vi "AFM_Driver_Manager.CreateAbort.vi"(8 "error in (no error)":errorcluster, 11 "AFM_Driver_Manager in":refnum<class "AFM_Driver_Manager.lvclass">) -> (0 "error out":errorcluster, 3 "AFM_Driver_Manager out":refnum<class "AFM_Driver_Manager.lvclass">)   [LabVIEW 2019, in "AFM_Driver_Manager.lvclass"]
uses:
  AFM_Driver_Manager.lvclass
  AFM_Driver_Manager.lvclass/AFM_Driver_Manager.ctl
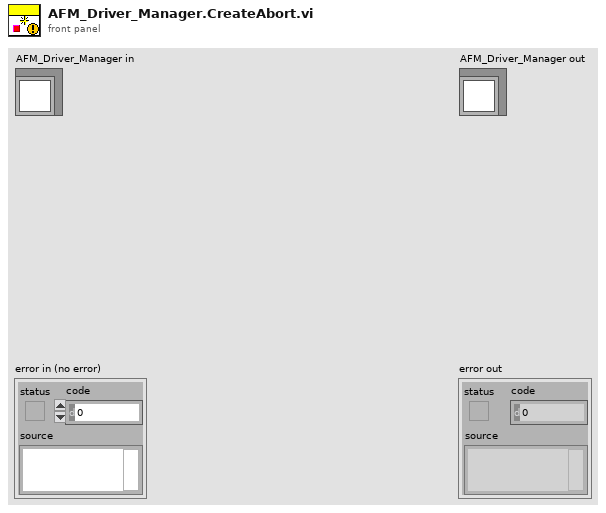
[diagram p1: front panel]
types:
  T1 = typedef "AFM_Driver_Manager.lvclass/AFM_Driver_Manager.PublicMethods.ctl" = cluster{"Stop Event":refnum<user-event>, "Lithography Data":refnum<user-event>, "Run Lithography":refnum<user-event>, "Background Image":refnum<user-event>, "Abort Notifier":refnum<user-event>}
  T2 = cluster{"VI Refnum":refnum<vi>, "Path":path, "Name":string, "Events":T1}
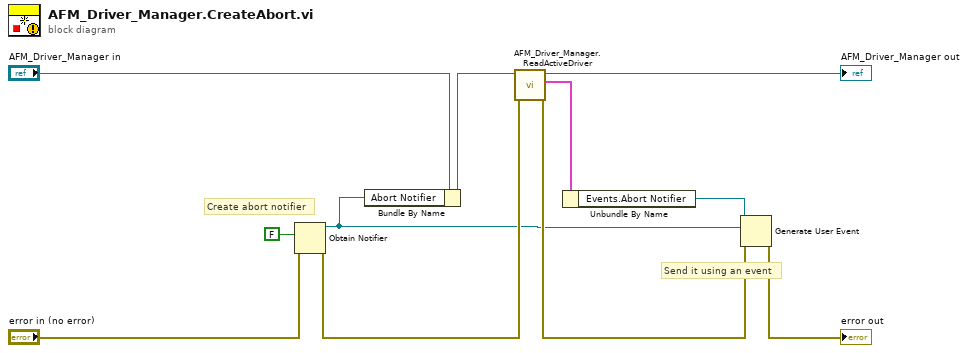
[diagram p0: block diagram]
diagram:
  # "Send it using an event"
  # "Create abort notifier"
  n1 = Obtain Notifier(notification data type=FALSE, error in (no error)="error in (no error)") -> (notifier out=w2:refnum<notifier>, error out=w6:errorcluster)  [unwired: 2 in, 1 out]
  n2 = Bundle By Name(cluster="AFM_Driver_Manager in", "Abort Notifier"=w2) -> (w4:refnum<class "AFM_Driver_Manager.lvclass">)
  n3 = call "AFM_Driver_Manager.ReadActiveDriver.vi"("error in (no error)"=w6, "AFM_Driver_Manager in"=w4) -> ("error out"=w5:errorcluster, "Active Driver"=w8:T2, "AFM_Driver_Manager out"=→"AFM_Driver_Manager out":refnum<class "AFM_Driver_Manager.lvclass">)  [unwired: 7 in]
  n4 = Unbundle By Name(w8) -> ("Events.Abort Notifier"=w1:refnum<user-event>)
  n5 = Generate User Event(user event=w1, event data cluster=w2, error in=w5) -> (error out=→"error out":errorcluster)  [unwired: 1 in, 1 out]
